vi "GetAvgPatientStayTimeSingleRoom.vi"(8 "error in":errorcluster, 9 "To":timestamp, 10 "From":timestamp, 11 "RoomNumber":string) -> (0 "error out":errorcluster, 1 "AvgStayTime(s)":dbl, 2 "PatientStayTime(s)":dbl[](array[numeric]), 3 "NumOfPatients":i32)   [LabVIEW 2015, in "DatabaseApi.lvlib"]
uses:
  DatabaseApi.lvlib
  TypeDef/Room/RoomFilter.ctl
  TypeDef/Room/RoomTableFilterRing.ctl
  LVClasses/Flags/ColorFlags.ctl
  LVClasses/Flags/ColorEnum.ctl
  LVClasses/Flags/Flags.lvclass
panel:
  out "Array 3":u32[](array[numeric])
  out "Array 2":T1(array[ring])
  out "Array":bool[](array[boolean])
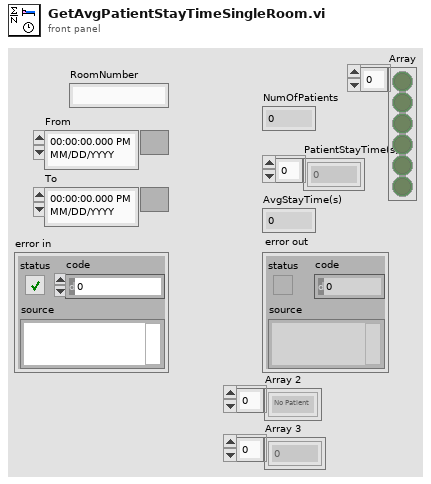
[diagram p1: front panel]
types:
  T1 = enum16{"No Patient", "Patient Admitted", "Patient Released", "Patient In Room"}[]
  T2 = typedef "DatabaseApi.lvlib/RoomTableFilterRing.ctl" = enum16{"Room Number", "Event Time", "Flags", "Bed Vacant", "In Room Personnel"}
  T3 = typedef "DatabaseApi.lvlib/RoomFilter.ctl" = cluster{"Filter":T2, "From":timestamp, "To":timestamp, "Filter Text":string, "RoomNumFlags":T4, "BedVacant":bool, "Enable Filter":bool}
  T4 = typedef "Flags.lvclass/ColorFlags.ctl" = cluster{"Flag State":u8[]}
  T5 = enum16{"No Patient", "Patient Admitted", "Patient Released", "Patient In Room"}
  T6 = typedef "Flags.lvclass/ColorEnum.ctl" = enum8{"Red", "Blue", "Green", "Yellow"}
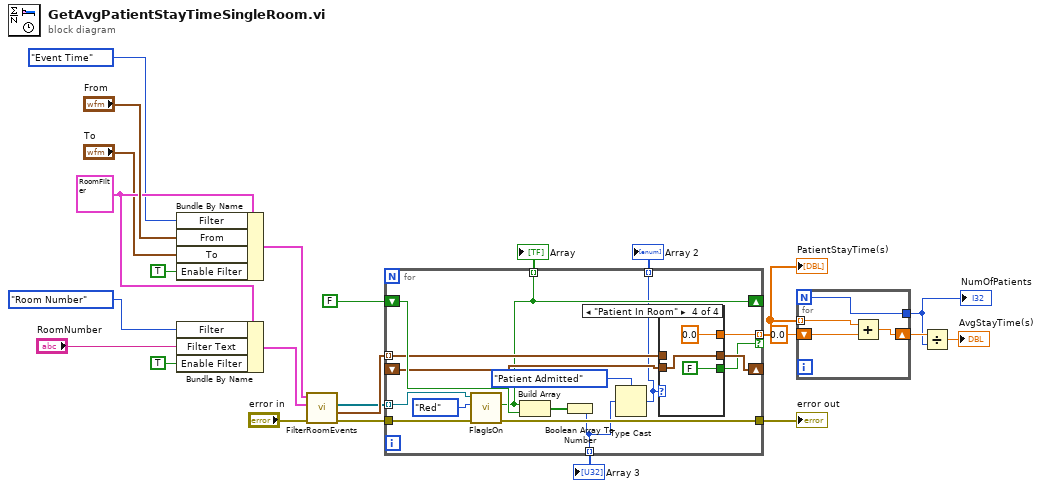
[diagram p0: block diagram]
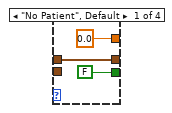
[diagram p2: hidden frame]
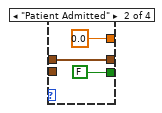
[diagram p3: hidden frame]
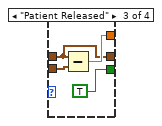
[diagram p4: hidden frame]
diagram:
  w22 = T3 {"Filter"=enum."Flags", "From"=timestamp(0 s since 1904-01-01), "To"=timestamp(0 s since 1904-01-01), "Filter Text"="", "RoomNumFlags"={"Flag State"=[1, 3, 5, 7]}, "BedVacant"=FALSE, "Enable Filter"=FALSE} ("Filter")
  n1 = Bundle By Name(cluster=w22, "Filter"=RoomTableFilterRing."Event Time", "From"="From", "To"="To", "Enable Filter"=TRUE) -> (w14:T3)
  n2 = Bundle By Name(cluster=w22, "Filter"=RoomTableFilterRing."Room Number", "Filter Text"="RoomNumber", "Enable Filter"=TRUE) -> (w13:T3)
  n3 = call "FilterRoomEvents.vi"("error in"="error in", "Filter 2"=w13, "Filter 1"=w14) -> ("error out"=w12:errorcluster, "EventTimeArray"=w15:timestamp[], "RoomArray"=w7:refnum<class "Room.lvclass">[])  [unwired: 6 in]
  n4 = for {
    tunnel: w7 -> [w38] mode=indexing
    tunnel: w15 -> [w31] mode=indexing
    tunnel: w12 -> [w39]
    tunnel: [w37] -> w6
    shift-right: [w27] -> _
    shift-left: FALSE -> [w35]
    shift-right: [w32] -> _
    shift-left: _ -> [w30]
    tunnel: [w29] -> w5 mode=indexing if=w28
    tunnel: [w27] -> w4 mode=indexing
    tunnel: [w26] -> w3 mode=indexing
    tunnel: [w25] -> w2 mode=indexing
    n5 = call "FlagIsOn.vi"("error in (no error)"=w39, "Flag to Check"=ColorEnum."Red", "Room in"=w38) -> ("error out"=w37:errorcluster, "Flag Is On"=w27:bool)  [unwired: 7 in]
    n6 = Build Array(w27, w35) -> (w34:bool[])
    n7 = Boolean Array To Number(Boolean array=w34) -> (number=w25:u16)
    n8 = Type Cast(type=T5."Patient Admitted", x=w25) -> (*(type *) &x=w26:T5)
    n9 = case shown="\"Patient In Room\"" w26 {
      tunnel: [w41 w45 w46 w51] -> w32
      tunnel: w31 -> [w41 w45 w46 _]
      tunnel: w30 -> [_ _ w49 w51]
      tunnel: [0.0 0.0 w48 0.0] -> w29
      tunnel: [FALSE FALSE TRUE FALSE] -> w28
      frame "No Patient", Default {
      }
      frame "Patient Admitted" {
      }
      frame "Patient Released" {
        n10 = Subtract(x=w46, y=w49) -> (x-y=w48:dbl)
      }
      frame "Patient In Room" {
      }
    }
  }
  "error out" <- w6
  "PatientStayTime(s)" <- w5
  "Array" <- w4
  "Array 2" <- w3
  "Array 3" <- w2
  n11 = for {
    N -> [w53]
    tunnel: w5 -> [w56] mode=indexing
    shift-right: [w55] -> w10
    shift-left: 0.0 -> [w54]
    tunnel: [w53] -> w8
    n12 = Add(x=w56, y=w54) -> (x+y=w55:dbl)
  }
  "NumOfPatients" <- w8
  n13 = Divide(x=w10, y=w8) -> (x/y=→"AvgStayTime(s)":dbl)
